vi "NI VeriStand - Get Item Data.vi"(8 "error in (no error)":errorcluster, 11 "Item Ref in":T2 format="%.0x") -> (0 "error out":errorcluster, 2 "Item Info":T1, 3 "Item Ref out":T2 format="%.0x", 4 "Found":bool)   [LabVIEW 2019, in "Custom Device API.lvlib"]
doc: "Returns information about the custom device item specified by <B>Item Ref in</B>, including the name of the item, the GUID of the associated configuration page, and whether the item is a channel."
uses:
  Custom Device API.lvlib
  Custom Device Item Ref.ctl
  Custom Device Item Info.ctl
  Custom Device Offline Path.vi
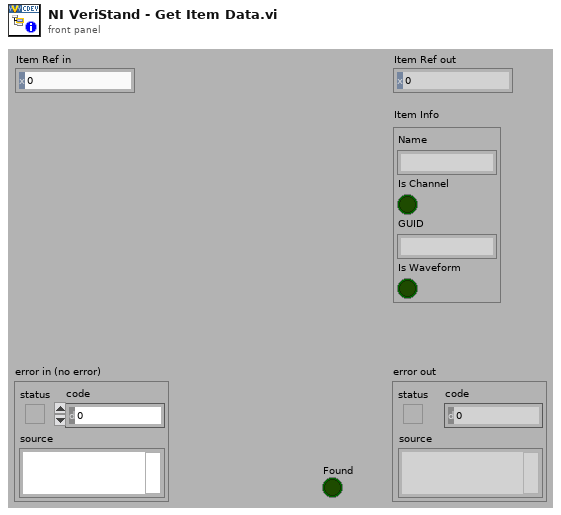
[diagram p1: front panel]
types:
  T1 = typedef "Custom Device API.lvlib/Custom Device Item Info.ctl" = cluster{"Name":string, "Is Channel":bool, "GUID":string, "Is Waveform":bool}
  T2 = typedef "Custom Device API.lvlib/Custom Device Item Ref.ctl" = u64
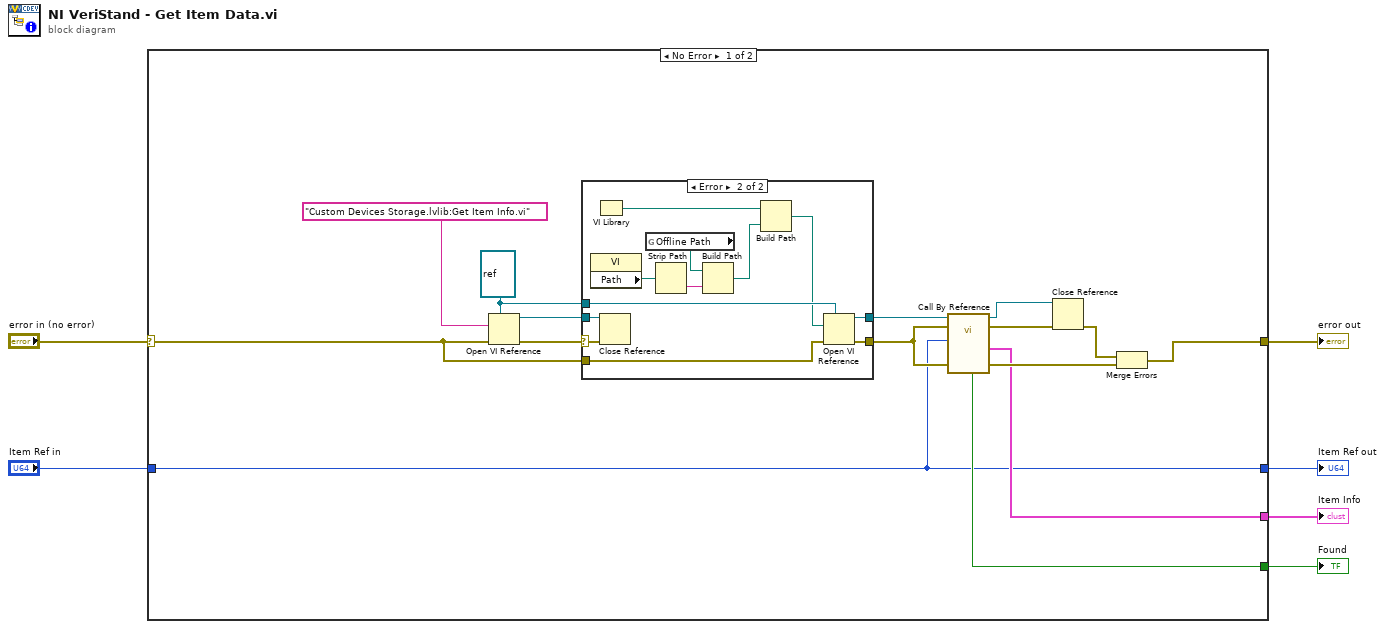
[diagram p0: block diagram]
diagram:
  n1 = case shown="No Error" "error in (no error)" {
    selector: "error in (no error)" -> [w16 w37]
    tunnel: [w20 w37] -> w6
    tunnel: "Item Ref in" -> [w15 w36]
    tunnel: [w15 w36] -> w4
    tunnel: [w19 _] -> w3
    tunnel: [w18 _] -> w2
    frame No Error {
      w9 = refnum<vi> refnum ("type specifier VI Refnum (for type only)")
      n2 = Open VI Reference(type specifier VI Refnum (for type only)=w9, vi path="Custom Devices Storage.lvlib:Get Item Info.vi", error in (no error)=w16) -> (vi reference=w10:refnum<vi>, error out=w11:errorcluster)  [unwired: 3 out]
      n3 = case shown="Error" w11 {
        selector: w11 -> [w22 w32]
        tunnel: w9 -> [_ w34]
        tunnel: w10 -> [w23 w33]
        tunnel: [w23 w31] -> w13
        tunnel: [w22 w30] -> w17
        tunnel: w16 -> [_ w35]
        frame No Error {
        }
        frame Error {
          n4 = property class="VI"() -> ("Path"=w25:path)  [unwired: 2 in, 2 out]
          n5 = VI Library() -> (path=w29:path)
          n6 = Close Reference(reference=w33, error in (no error)=w32) -> ()  [unwired: 1 out]
          n7 = global read "Custom Device Offline Path.vi" "Offline Path"() -> (w26:path)
          n8 = Strip Path(path=w25) -> (name=w24:string)  [unwired: 1 out]
          n9 = Build Path(base path=w26, name or relative path=w24) -> (appended path=w28:path)
          n10 = Build Path(base path=w29, name or relative path=w28) -> (appended path=w27:path)
          n11 = Open VI Reference(type specifier VI Refnum (for type only)=w34, vi path=w27, error in (no error)=w35) -> (vi reference=w31:refnum<vi>, error out=w30:errorcluster)  [unwired: 3 out]
        }
      }
      n12 = call-by-ref "?"(reference=w13, error in=w17, 8:"error in (no error)"=w17, "Item Ref in"=w15) -> (reference out=w7:refnum<vi>, error out=w14:errorcluster, 0:"error out"=w21:errorcluster, "Item Info"=w19:T1, "Found"=w18:bool)  [unwired: 6 in, 1 out]
      n13 = Close Reference(reference=w7, error in (no error)=w14) -> (error out=w8:errorcluster)
      n14 = Merge Errors(w8, w21) -> (w20:errorcluster)
    }
    frame Error {
    }
  }
  "Item Ref out" <- w4
  "error out" <- w6
  "Found" <- w2
  "Item Info" <- w3
